vi "Update Online Status.vi"(8 "error in (no error)":errorcluster, 11 "Chat Window Controller in":refnum<class "Chat Window Controller.lvclass">) -> (0 "error out":errorcluster, 3 "Chat Window Controller out":refnum<class "Chat Window Controller.lvclass">)   [LabVIEW 2020, in "Chat Window Controller.lvlib" / "Chat Window Controller.lvclass"]
uses:
  Chat Window Controller.lvclass
  Chat Window Controller.lvclass/Chat Window Controller.ctl
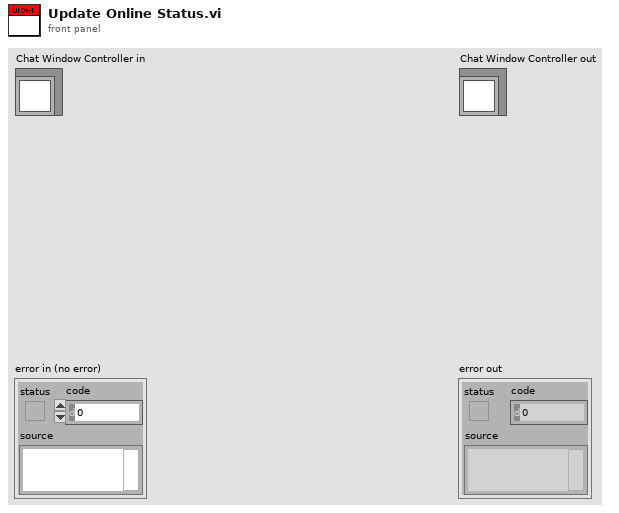
[diagram p1: front panel]
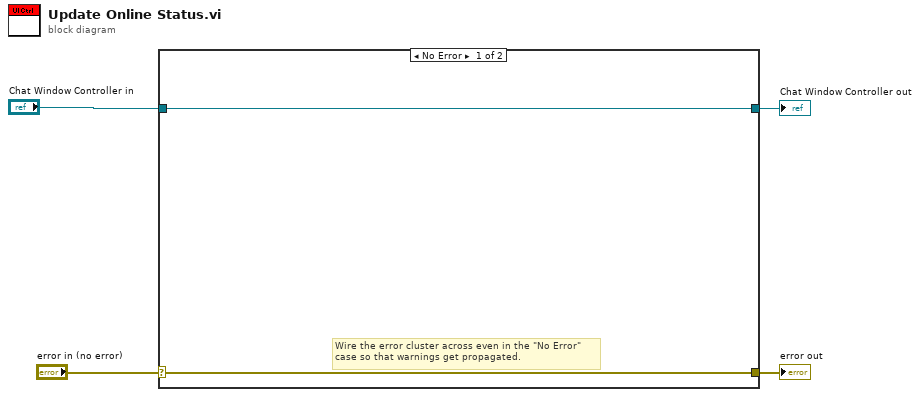
[diagram p0: block diagram]
diagram:
  n1 = case shown="No Error" "error in (no error)" {
    selector: "error in (no error)" -> [w5 w8]
    tunnel: [w5 w8] -> w3
    tunnel: [w6 w7] -> w1
    tunnel: "Chat Window Controller in" -> [w6 w7]
    frame No Error {
      # "Wire the error cluster across even in the \"No Error\"\ncase so that warnings get propagated."
    }
    frame Error {
    }
  }
  "error out" <- w3
  "Chat Window Controller out" <- w1
